vi "p1.vi"() -> ()   [LabVIEW 2023, in "d25.lvlib"]
uses:
  d25.lvlib
  AOC/AOC.lvlib
panel:
  out "SNAFU":string
  in  "Example":string="1=-0-2\n12111\n2=0=\n21\n2=01\n111\n20012\n112\n1=-1=\n1-12\n12\n1=\n122"
  in  "Example":bool
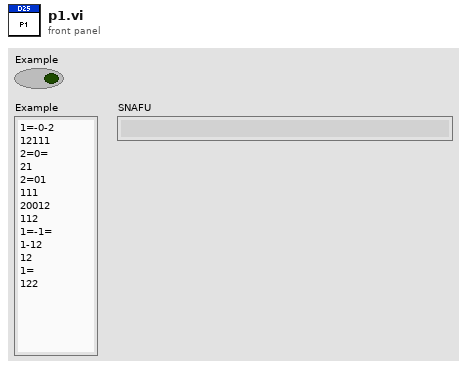
[diagram p1: front panel]
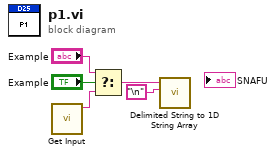
[diagram p0: block diagram]
diagram:
  n1 = call "Get Input.vi"() -> ("Input"=w5:string)  [unwired: 11 in]
  n2 = Select(t="Example", s="Example", f=w5) -> (s? t:f=w4:string)
  n3 = call <vilib>:"Delimited String to 1D String Array.vi"("delimiter"="\n", "delimited string"=w4) -> ()  [unwired: 9 in, 1 out]
